vi "Write Header.vi"(8 "Error In":errorcluster, 9 "Module Init Timestamp":timestamp, 10 "Application Name":string, 11 "File refnum":refnum<file>) -> (0 "Error Out":errorcluster)   [LabVIEW 2023, in "Error Manager.lvlib" / "Error Log.lvclass"]
uses:
  Error Log.lvclass
  Error Log.lvclass/Error Log.ctl
  Error Manager.lvlib
panel:
  out "Text written to log":string
  # "Input\nInputs to the VI"
  # "Development\nControls or indicators that are useful for development or testing, but which are not outputs of the VI."
  # "Output\nOutputs of the VI"
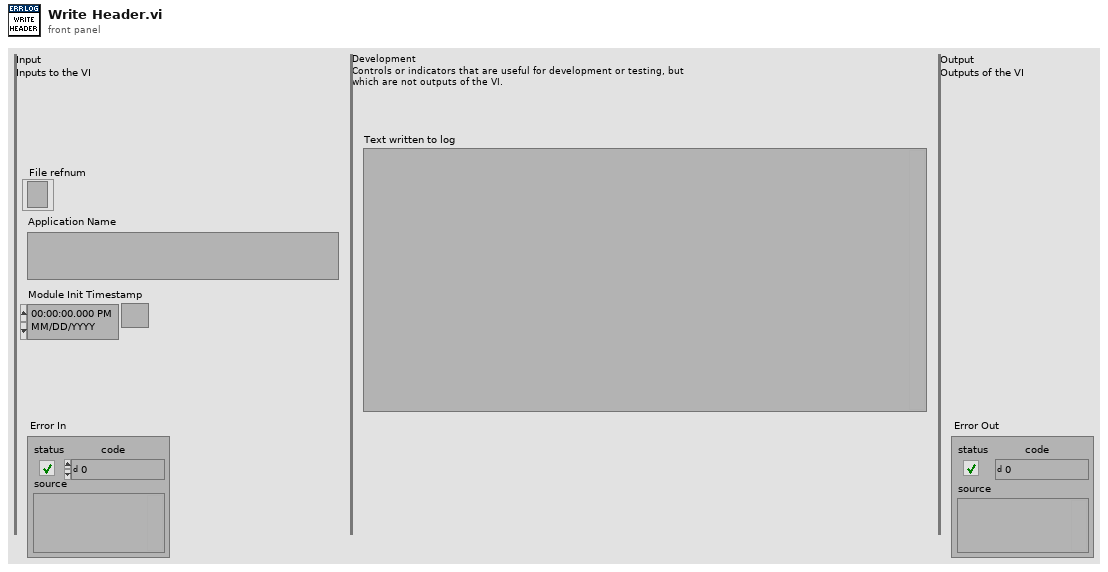
[diagram p1: front panel]
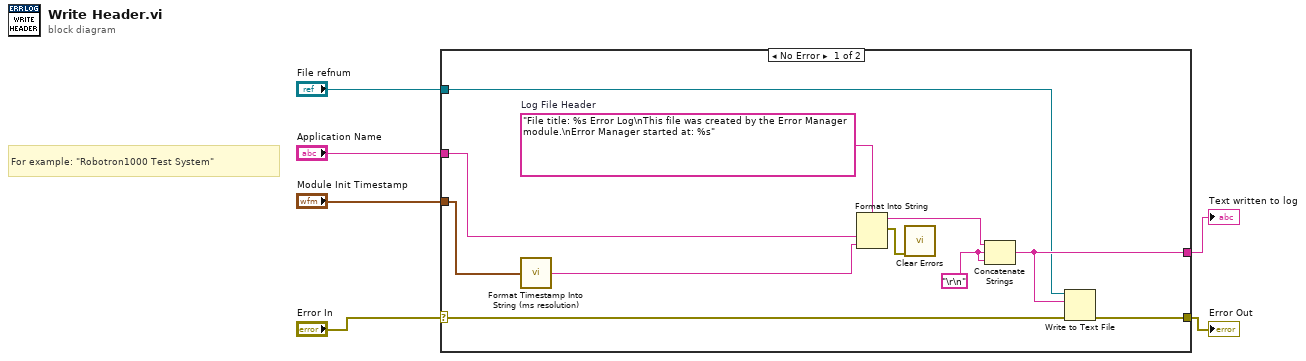
[diagram p0: block diagram]
diagram:
  # "For example: \"Robotron1000 Test System\""
  n1 = case shown="No Error" "Error In" {
    selector: "Error In" -> [w16 w18]
    tunnel: [w17 w18] -> w5
    tunnel: "Module Init Timestamp" -> [w8 _]
    tunnel: "Application Name" -> [w12 _]
    tunnel: [w11 _] -> w2
    tunnel: "File refnum" -> [w10 _]
    frame No Error {
      w13 = "\r\n"
      w15 = "File title: %s Error Log\nThis file was created by the Error Manager module.\nError Manager started at: %s"  # Log File Header
      n2 = call "Format Timestamp Into String (ms resolution).vi"("Timestamp"=w8) -> ("Timestamp String (ms resolution)"=w7:string)
      n3 = Format Into String(format string=w15, w12, w7) -> (resulting string=w14:string, error out=w9:errorcluster)  [unwired: 2 in]
      n4 = call <vilib>:"Clear Errors.vi"("error in (no error)"=w9) -> ()  [unwired: 5 in, 2 out]
      n5 = Concatenate Strings(w14, w13, w13) -> (w11:string)
      n6 = Write to Text File(file (use dialog)=w10, text=w11, error in=w16) -> (error out=w17:errorcluster)  [unwired: 1 in, 2 out]
    }
    frame Error {
    }
  }
  "Error Out" <- w5
  "Text written to log" <- w2
